vi "Event New SW.vi"(8 "error in (no error)":errorcluster, 11 "[MV] Key Generator in":refnum<class "[MV] Key Generator.lvclass">) -> (0 "error out":errorcluster, 3 "[MV] Key Generator out":refnum<class "[MV] Key Generator.lvclass">)   [LabVIEW 2023, in "[MV] Key Generator.lvlib" / "[MV] Key Generator.lvclass"]
uses:
  [MV] Key Generator.lvclass
  [MV] Key Generator.lvclass/[MV] Key Generator.ctl
  <vilib>/YU/YU_Encrypt/RSA/RSA.lvclass
  <vilib>/YU/YU_Encrypt/Base64/Base64.lvclass
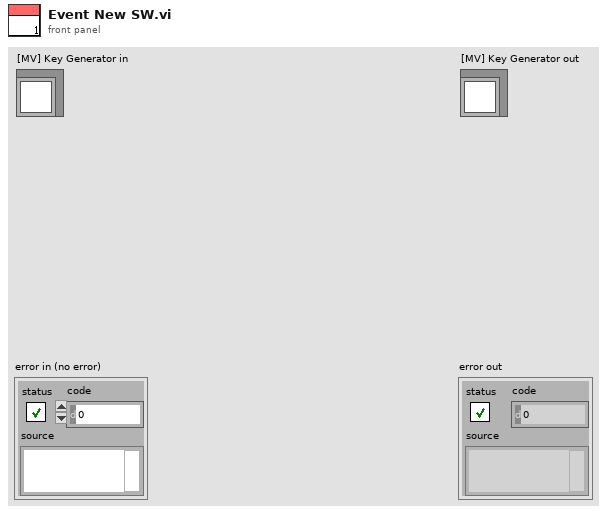
[diagram p1: front panel]
types:
  T1 = map{string, cluster{"private":string, "public":string}}
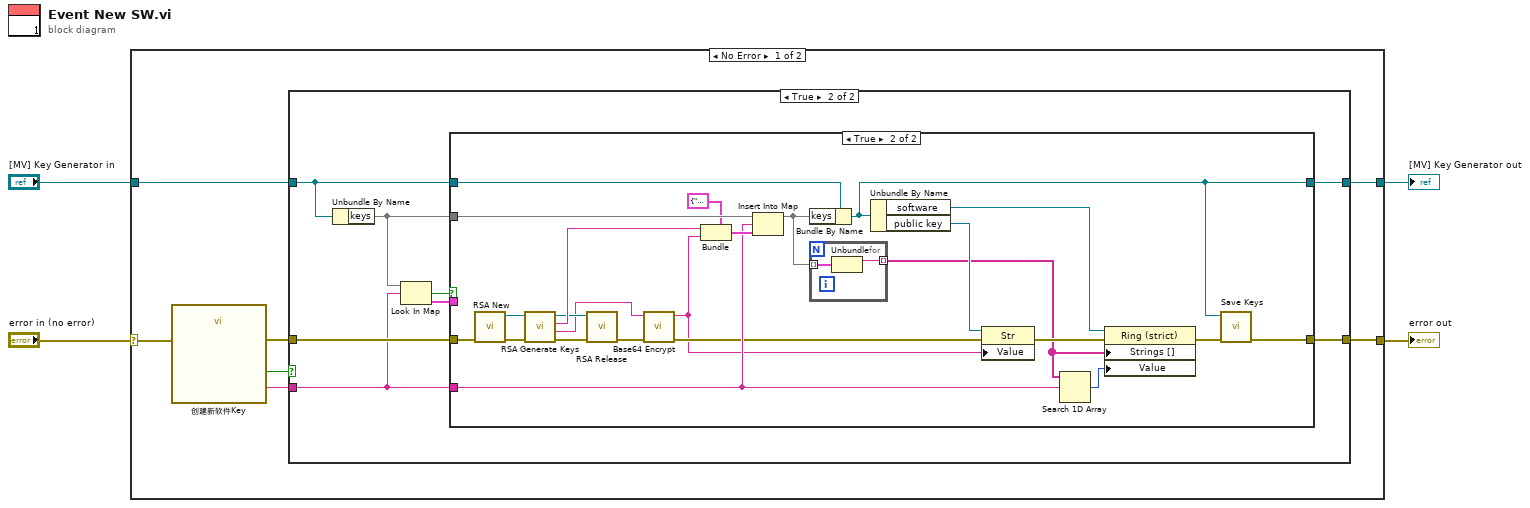
[diagram p0: block diagram]
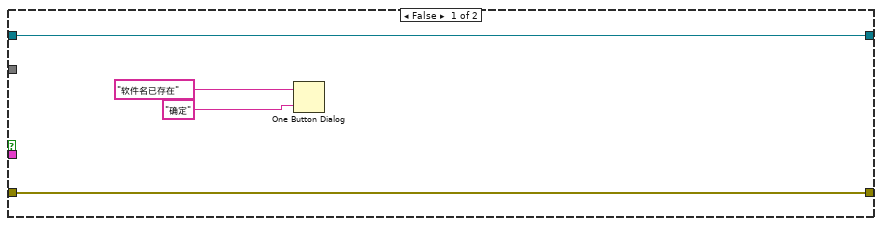
[diagram p3: hidden frame]
diagram:
  n1 = case shown="No Error" "error in (no error)" {
    selector: "error in (no error)" -> [w11 w53]
    tunnel: [w7 w53] -> w3
    tunnel: [w5 w52] -> w1
    tunnel: "[MV] Key Generator in" -> [w6 w52]
    frame No Error {
      n2 = call "创建新软件Key"("error in (no error)"=w11) -> ("软件名称"=w9:string, "确定"=w10:bool, "error out"=w8:errorcluster)  [unwired: 16 in]
      n3 = case shown="True" w10 {
        tunnel: w9 -> [_ w15]
        tunnel: w8 -> [w12 w19]
        tunnel: [w12 w17] -> w7
        tunnel: w6 -> [w13 w18]
        tunnel: [w13 w14] -> w5
        frame False {
        }
        frame True {
          n4 = Unbundle By Name(w18) -> ("keys"=w16:T1)
          n5 = Look In Map(map=w16, key=w15) -> (key not found?=w21:bool, value=w20:cluster{"private":string, "public":string})  [unwired: 1 in]
          n6 = case shown="True" w21 {
            tunnel: w20 -> [_ _]
            tunnel: w19 -> [w23 w49]
            tunnel: w18 -> [w22 w43]
            tunnel: [w23 w37] -> w17
            tunnel: w16 -> [_ w45]
            tunnel: w15 -> [_ w34]
            tunnel: [w22 w36] -> w14
            frame False {
              n7 = One Button Dialog(message="软件名已存在", button name ("OK")="确定") -> ()  [unwired: 1 out]
            }
            frame True {
              n8 = call <vilib>:"RSA New.vi"("error in (no error)"=w49) -> ("error out"=w48:errorcluster, "RSA out"=w47:refnum<class "RSA.lvclass">)  [unwired: 9 in]
              n9 = call <vilib>:"RSA Generate Keys.vi"("error in (no error)"=w48, "RSA in"=w47) -> ("error out"=w32:errorcluster, "public_key"=w27:string, "private_key"=w46:string, "RSA out"=w31:refnum<class "RSA.lvclass">)  [unwired: 6 in]
              n10 = call <vilib>:"RSA Release.vi"("error in (no error)"=w32, "RSA in"=w31) -> ("error out"=w30:errorcluster)  [unwired: 9 in]
              n11 = call <vilib>:"Base64 Encrypt.vi"("error in (no error)"=w30, "message"=w27) -> ("error out"=w29:errorcluster, "message_encrypted"=w26:string)  [unwired: 8 in]
              n12 = Bundle(cluster=cluster{"private":string, "public":string} {"private"="", "public"=""} ("key"), "private"=w46, "public"=w26) -> (w44:cluster{"private":string, "public":string})
              n13 = Insert Into Map(map in=w45, key=w34, value=w44) -> (map out=w42:T1)  [unwired: 2 out]
              n14 = Bundle By Name(cluster=w43, "keys"=w42) -> (w36:refnum<class "[MV] Key Generator.lvclass">)
              n15 = for {
                tunnel: w42 -> [w51] mode=indexing
                tunnel: [w50] -> w35 mode=indexing
                n16 = Unbundle(w51) -> ("name"=w50:string)  [unwired: 1 out]
              }
              n17 = Unbundle By Name(w36) -> ("software"=w40:refnum<vi>, "public key"=w39:refnum<vi>)
              n18 = property class="Str"(reference=w39, error in=w29, "Value"=w26) -> (error out=w41:errorcluster)  [unwired: 1 out]
              n19 = Search 1D Array(1D array=w35, element=w34) -> (index of element=w33:i32)  [unwired: 1 in]
              n20 = property class="Ring (strict)"(reference=w40, error in=w41, "Strings []"=w35, "Value"=w33) -> (error out=w38:errorcluster)  [unwired: 1 out]
              n21 = call "Save Keys.vi"("error in (no error)"=w38, "[MV] Key Generator in"=w36) -> ("error out"=w37:errorcluster)  [unwired: 8 in, 1 out]
            }
          }
        }
      }
    }
    frame Error {
    }
  }
  "error out" <- w3
  "[MV] Key Generator out" <- w1
